vi "VisaReadExample1.vi"() -> ()   [LabVIEW 2016]
uses:
  <vilib>/Instr/_visa.llb/VISA Configure Serial Port (Instr).vi
panel:
  out "PULSE":dbl(knob) scale=0.0..200.0
  out "DEVICE READY":bool
  in  "VISA resource name":refnum<visa-resource-name>="COM3"
  out "O2 SAT":dbl
  out "PULSE":dbl
  in  "Upper Cut-Off":dbl=100.0
  in  "Lower Cut-Off":dbl=10.0
  in  "OK Button":bool
  out "Waveform Graph":dynamicdata(graph)
  in  "Array 2":dbl[](array[numeric])=array[6515 elements]
  in  "Array":dbl[](array[numeric])=array[6516 elements]
  out "substring 2":string="I"
  out "substring":string="126526"
  out "read buffer":string="I126526"
  in  "stop":bool
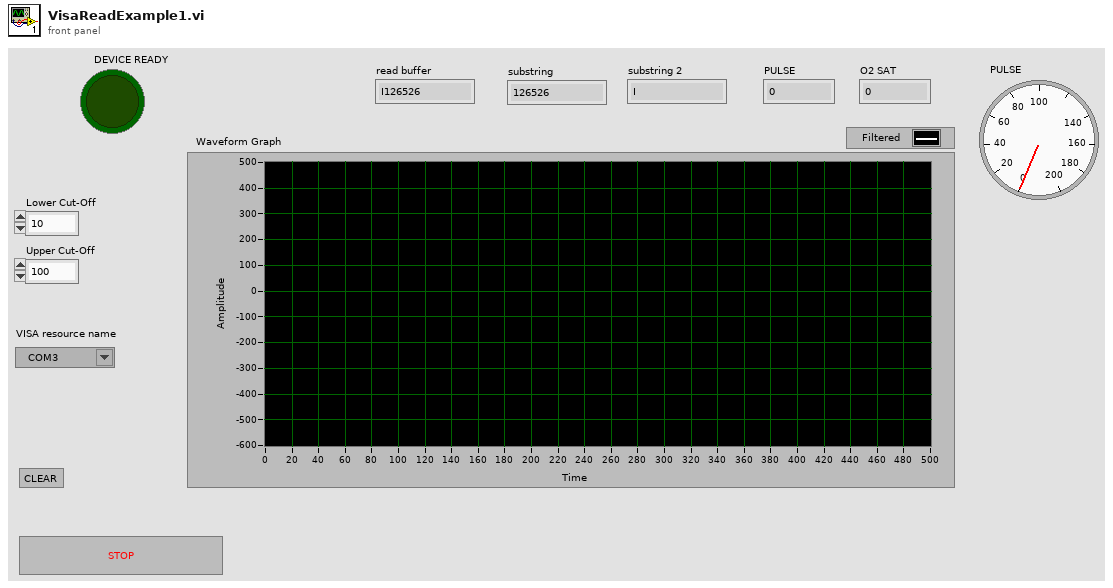
[diagram p1: front panel]
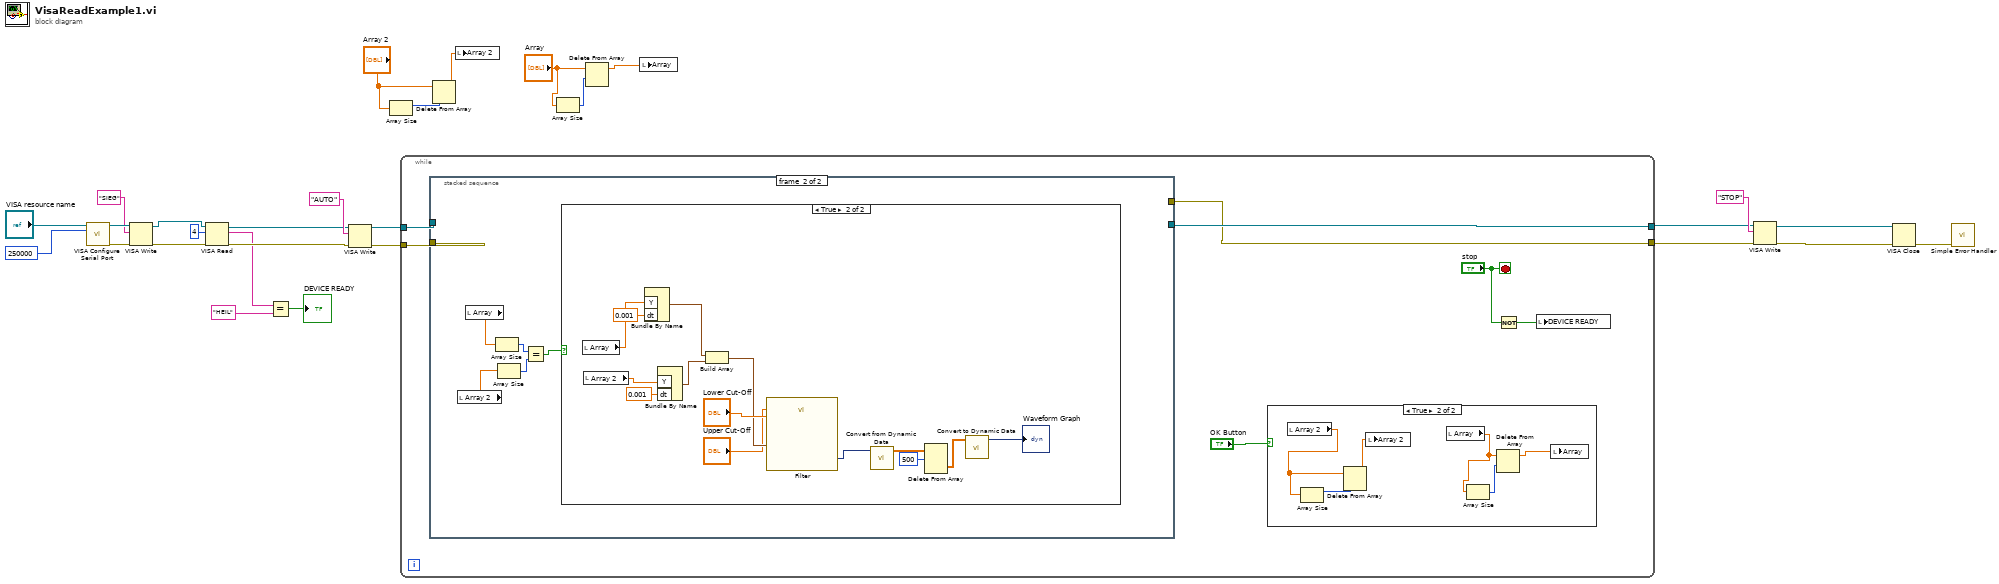
[diagram p0: block diagram]
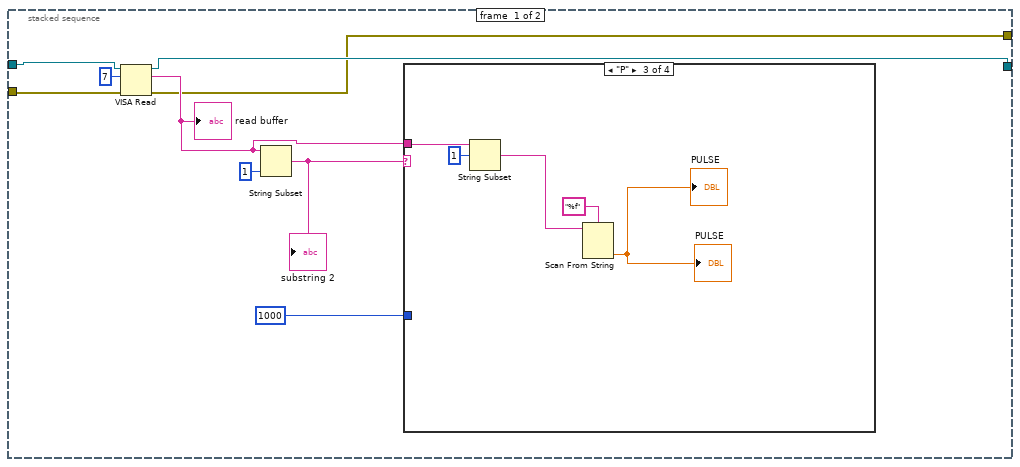
[diagram p3: hidden frame]
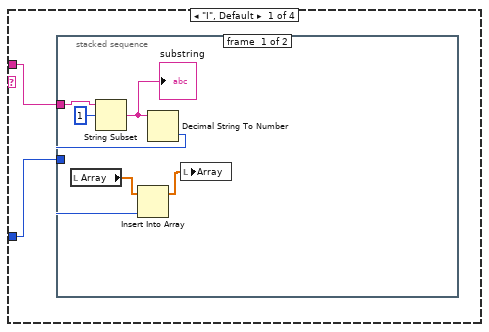
[diagram p4: hidden frame]
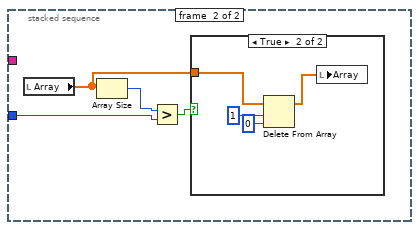
[diagram p5: hidden frame]
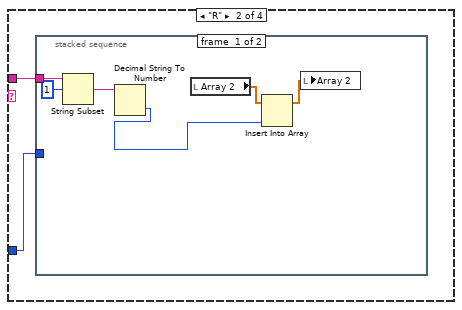
[diagram p7: hidden frame]
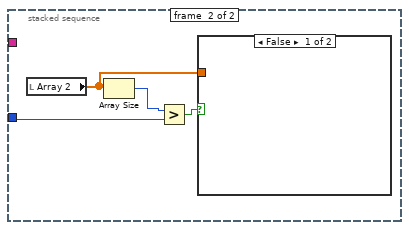
[diagram p8: hidden frame]
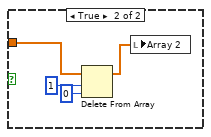
[diagram p9: hidden frame]
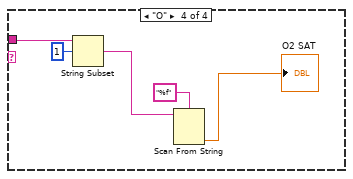
[diagram p10: hidden frame]
diagram:
  n1 = call-poly "VISA Configure Serial Port"("VISA resource name"="VISA resource name", "baud rate (9600)"=u32 250000) -> ("VISA resource name out"=w16:refnum<visa-resource-name>, "error out"=w15:errorcluster)  [unwired: 12 in]
  n2 = VISA Write(VISA resource name=w16, write buffer="SIEG", error in (no error)=w15) -> (VISA resource name out=w12:refnum<visa-resource-name>, error out=w11:errorcluster)  [unwired: 1 out]
  n3 = VISA Read(VISA resource name=w12, byte count=u32 4, error in (no error)=w11) -> (VISA resource name out=w9:refnum<visa-resource-name>, read buffer=w8:string, error out=w10:errorcluster)  [unwired: 1 out]
  n4 = Equal?(x=w8, y="HEIL") -> (x = y?=→"DEVICE READY":bool)
  n5 = VISA Write(VISA resource name=w9, write buffer="AUTO", error in (no error)=w10) -> (VISA resource name out=w27:refnum<visa-resource-name>, error out=w26:errorcluster)  [unwired: 1 out]
  n6 = Array Size(array="Array 2") -> (size(s)=w21:i32)
  n7 = while {
    tunnel: [w35] -> w3
    tunnel: w27 -> [w34]
    tunnel: w26 -> [w33]
    tunnel: [w31] -> w2
    stop <- "stop" stop-if-true
    n8 = stacked-sequence {
      tunnel: [w50 _] -> w35
      tunnel: w34 -> [w48 _]
      tunnel: w33 -> [w45 _]
      tunnel: [w42 _] -> w31
      frame #0 {
        n9 = VISA Read(VISA resource name=w48, byte count=u32 7, error in (no error)=w45) -> (VISA resource name out=w50:refnum<visa-resource-name>, read buffer=w44:string, error out=w42:errorcluster)  [unwired: 1 out]
        "read buffer" <- w44
        n10 = String Subset(string=w44, length (rest)=1 ("length (rest)")) -> (substring=w46:string)  [unwired: 1 in]
        "substring 2" <- w46
        n11 = case shown="\"P\"" w46 {
          tunnel: w44 -> [w52 w68 w86 w91]
          tunnel: 1000 ("y") -> [w51 w67 _ _]
          frame "I", Default {
            n12 = stacked-sequence {
              tunnel: w52 -> [w57 _]
              tunnel: w51 -> [_ w61]
              frame #0 {
                n13 = local read "Array"() -> (w55:dbl[])
                n14 = String Subset(string=w57, offset (0)=1) -> (substring=w56:string)  [unwired: 1 in]
                "substring" <- w56
                n15 = Decimal String To Number(string=w56) -> (number=w54:i32)  [unwired: 2 in, 1 out]
                n16 = Insert Into Array(array=w55, new element=w54) -> (w53:dbl[])  [unwired: 1 in]
                n17 = local write "Array"(w53) -> ()
              }
              frame #1 {
                n18 = local read "Array"() -> (w59:dbl[])
                n19 = Array Size(array=w59) -> (size(s)=w62:i32)
                n20 = Greater?(x=w62, y=w61) -> (0:w60:bool)
                n21 = case shown="True" w60 {
                  tunnel: w59 -> [_ w66]
                  frame False {
                  }
                  frame True {
                    n22 = Delete From Array(array=w66, length=1, index=0) -> (array with subset deleted=w63:dbl[])  [unwired: 1 out]
                    n23 = local write "Array"(w63) -> ()
                  }
                }
              }
            }
          }
          frame "R" {
            n24 = stacked-sequence {
              tunnel: w68 -> [w74 _]
              tunnel: w67 -> [_ w75]
              frame #0 {
                n25 = String Subset(string=w74, offset (0)=1) -> (substring=w72:string)  [unwired: 1 in]
                n26 = Decimal String To Number(string=w72) -> (number=w70:i32)  [unwired: 2 in, 1 out]
                n27 = local read "Array 2"() -> (w71:dbl[])
                n28 = Insert Into Array(array=w71, new element=w70) -> (w69:dbl[])  [unwired: 1 in]
                n29 = local write "Array 2"(w69) -> ()
              }
              frame #1 {
                n30 = local read "Array 2"() -> (w76:dbl[])
                n31 = Array Size(array=w76) -> (size(s)=w78:i32)
                n32 = Greater?(x=w78, y=w75) -> (0:w77:bool)
                n33 = case shown="False" w77 {
                  tunnel: w76 -> [_ w82]
                  frame False {
                  }
                  frame True {
                    n34 = Delete From Array(array=w82, length=1, index=0) -> (array with subset deleted=w79:dbl[])  [unwired: 1 out]
                    n35 = local write "Array 2"(w79) -> ()
                  }
                }
              }
            }
          }
          frame "P" {
            n36 = String Subset(string=w86, offset (0)=1) -> (substring=w84:string)  [unwired: 1 in]
            n37 = Scan From String(format string="%f", input string=w84) -> (output 1=→"PULSE" →"PULSE":dbl)  [unwired: 3 in, 3 out]
          }
          frame "O" {
            n38 = String Subset(string=w91, offset (0)=1) -> (substring=w88:string)  [unwired: 1 in]
            n39 = Scan From String(format string="%f", input string=w88) -> (output 1=→"O2 SAT":dbl)  [unwired: 3 in, 3 out]
          }
        }
      }
      frame #1 {
        n40 = local read "Array 2"() -> (w97:dbl[])
        n41 = local read "Array"() -> (w96:dbl[])
        n42 = Array Size(array=w96) -> (size(s)=w95:i32)
        n43 = Array Size(array=w97) -> (size(s)=w94:i32)
        n44 = Equal?(x=w95, y=w94) -> (x = y?=w93:bool)
        n45 = case shown="True" w93 {
          frame False {
          }
          frame True {
            n46 = local read "Array"() -> (w111:dbl[])
            n47 = local read "Array 2"() -> (w110:dbl[])
            n48 = Bundle By Name("Y"=w111, "dt"=0.001) -> (w106:waveform(dbl))  [unwired: 1 in]
            n49 = Bundle By Name("Y"=w110, "dt"=0.001) -> (w107:waveform(dbl))  [unwired: 1 in]
            n50 = Build Array(w106, w107) -> (w101:waveform(dbl)[])
            n51 = call "Filter"("Lower Cut-Off"="Lower Cut-Off", "Upper Cut-Off"="Upper Cut-Off", "Signal"=w101) -> ("Filtered Signal"=w100:dynamicdata)  [unwired: 7 in, 1 out]
            n52 = call "Convert from Dynamic Data"("Dynamic Data Type"=w100) -> ("Array"=w104:dbl[][])  [unwired: 3 in]
            n53 = Delete From Array(array=w104, length=500) -> (deleted portion=w99:dbl[][])  [unwired: 2 in, 1 out]
            n54 = call "Convert to Dynamic Data"("2D Array"=w99) -> ("Dynamic Data Type"=→"Waveform Graph":dynamicdata)  [unwired: 3 in]
          }
        }
      }
    }
    n55 = case shown="True" "OK Button" {
      frame False {
      }
      frame True {
        n56 = local read "Array 2"() -> (w37:dbl[])
        n57 = Array Size(array=w37) -> (size(s)=w40:i32)
        n58 = Delete From Array(array=w37, length=w40) -> (array with subset deleted=w39:dbl[])  [unwired: 1 in, 1 out]
        n59 = local write "Array 2"(w39) -> ()
        n60 = local read "Array"() -> (w36:dbl[])
        n61 = Array Size(array=w36) -> (size(s)=w41:i32)
        n62 = Delete From Array(array=w36, length=w41) -> (array with subset deleted=w38:dbl[])  [unwired: 1 in, 1 out]
        n63 = local write "Array"(w38) -> ()
      }
    }
    n64 = Not(x="stop") -> (.not. x?=w30:bool)
    n65 = local write "DEVICE READY"(w30) -> ()
  }
  n66 = Delete From Array(array="Array 2", length=w21) -> (array with subset deleted=w23:dbl[])  [unwired: 1 in, 1 out]
  n67 = local write "Array 2"(w23) -> ()
  n68 = Array Size(array="Array") -> (size(s)=w19:i32)
  n69 = Delete From Array(array="Array", length=w19) -> (array with subset deleted=w24:dbl[])  [unwired: 1 in, 1 out]
  n70 = local write "Array"(w24) -> ()
  n71 = VISA Write(VISA resource name=w3, write buffer="STOP", error in (no error)=w2) -> (VISA resource name out=w4:refnum<visa-resource-name>, error out=w5:errorcluster)  [unwired: 1 out]
  n72 = VISA Close(VISA resource name=w4, error in (no error)=w5) -> (error out=w28:errorcluster)
  n73 = call <vilib>:"Simple Error Handler.vi"("error in (no error)"=w28) -> ()  [unwired: 4 in, 5 out]
